vi "PR_Update_spout_time  .vi"(8 "error in (no error)":errorcluster, 10 "barcode":string="123465798", 11 "DBlink":string="Driver={ODBC Driver 17 for SQL Server};Server=localhost\\SQLEXPRESS;Database=ZDX201;UID=labview;PWD=Dsa@54137926") -> (0 "error out":errorcluster)   [LabVIEW 2019]
uses:
  <vilib>/addons/database/Connection.llb/DB Tools Open Connec (String).vi
  <vilib>/addons/database/NI_Database_API.lvlib
panel:
  out "concatenated string":string="WHERE [barcode]='984132195' and [pos]='B'"
  in  "columns":string[](array[string])=["[time_spout]", "update_time"]
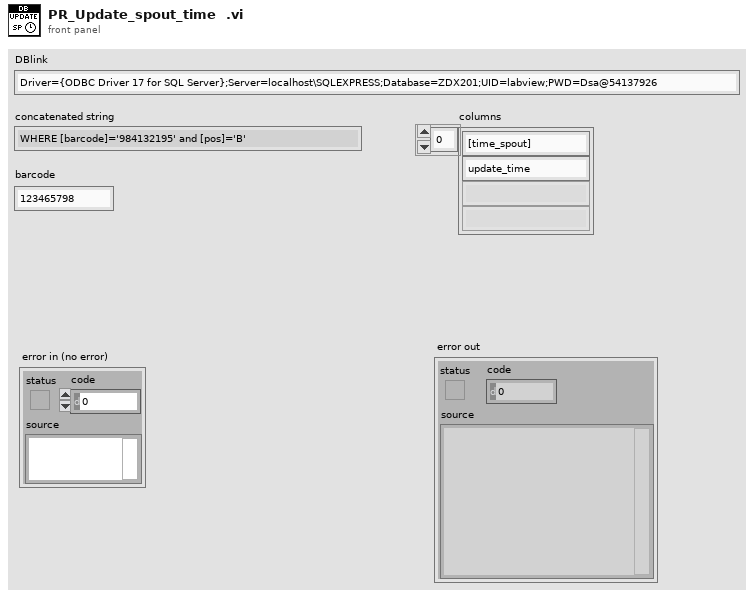
[diagram p1: front panel]
types:
  T1 = cluster{"[time_spout]":timestamp, "update_time":timestamp}
  T2 = typedef "NI_Database_API.lvlib/Conn ObjectReference.ctl" = refnum<k1>
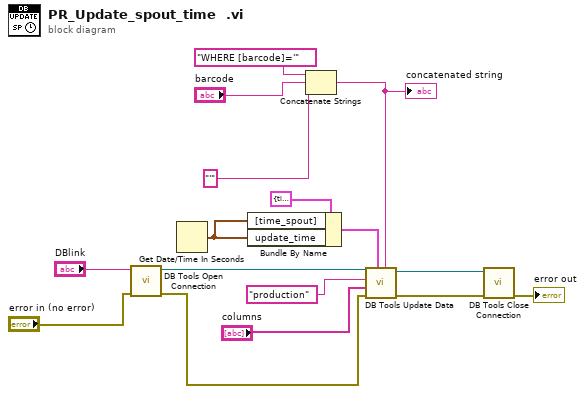
[diagram p0: block diagram]
diagram:
  n1 = call-poly <vilib>:"DB Tools Open Connection.vi"("error in (no error)"="error in (no error)", "connection information"="DBlink") -> ("error out"=w14:errorcluster, "connection reference"=w12:T2)  [unwired: 6 in]
  n2 = Get Date/Time In Seconds() -> (seconds since 1Jan1904=w2:timestamp)
  n3 = Bundle By Name(cluster=T1 {"[time_spout]"=timestamp(0 s since 1904-01-01), "update_time"=timestamp(0 s since 1904-01-01)}, "[time_spout]"=w2, "update_time"=w2) -> (w1:T1)
  n4 = Concatenate Strings("WHERE [barcode]='", "barcode", "'" ("string")) -> (w6:string)
  "concatenated string" <- w6
  n5 = call <vilib>:"DB Tools Update Data.vi"("condition"=w6, "data"=w1, "error in (no error)"=w14, "columns"="columns", "table"="production", "connection reference"=w12) -> ("error out"=w15:errorcluster, "connection reference out"=w13:T2)  [unwired: 4 in]
  n6 = call <vilib>:"DB Tools Close Connection.vi"("error in (no error)"=w15, "connection reference"=w13) -> ("error out"=→"error out":errorcluster)  [unwired: 5 in]
